vi "Fetch Multi Eval Meas List IEM Margin Results.vi"(8 "error in (no error)":errorcluster, 9 "Result Type (Current)":i32(ring) items=["Current", "Average", "Extreme", "Standard Deviation"], 10 "Instance (1)":T2=1, 11 "VISA resource name":refnum<visa-resource-name>) -> (0 "error out":errorcluster, 1 "IEM Margin Results":T1(array[cluster]) {"Carrier Leakage" format="%^.3e"; "IQ Image" format="%^.3e"; "Margin" format="%^.3e"}, 2 "Reliability":i32, 3 "VISA resource name out":refnum<visa-resource-name>)   [LabVIEW 2020, in "Rohde&Schwarz CMXP NR FR2 Measurement.lvlib"]
doc: "Returns the inband emission limit line margin results for all measured list mode segments.\n\nAttributes:\nRSCMXPNRFR2M_ATTR_FETCH_MULTI_EVAL_MEASUREMENT_LIST_IEM_MARGIN_AVERAGE_RESULTS\nRSCMXPNRFR2M_ATTR_FETCH_MULTI_EVAL_MEASUREMENT_LIST_IEM_MARGIN_CURRENT_RESULTS\nRSCMXPNRFR2M_ATTR_FETCH_MULTI_EVAL_MEASUREMENT_LIST_IEM_MARGIN_EXTREME_RESULTS\nRSCMXPNRFR2M_ATTR_FETCH_MULTI_EVAL_MEASUREMENT_LIST_IEM_MARGIN_STANDARD_DEVIATION_RESULTS\n\nRemote-control commands:\nFETCh:NRMMw:MEAS<i>:MEValuation:LIST:IEMission:MARGin:AVERage?\nFETCh:NRMMw:MEAS<i>:MEValuation:LIST:IEMission:MARGin:CURRent?\nFETCh:NRMMw:MEAS<i>:MEValuation:LIST:IEMission:MARGin:EXTReme?\nFETCh:NRMMw:MEAS<i>:MEValuation:LIST:IEMission:MARGin:SDEViation?"
uses:
  <instrlib>/Rohde&Schwarz CMXP NR FR2 Measurement/Rohde&Schwarz CMXP NR FR2 Measurement.lvlib
  <instrlib>/Rohde&Schwarz CMXP NR FR2 Measurement/Private/_Instance.ctl
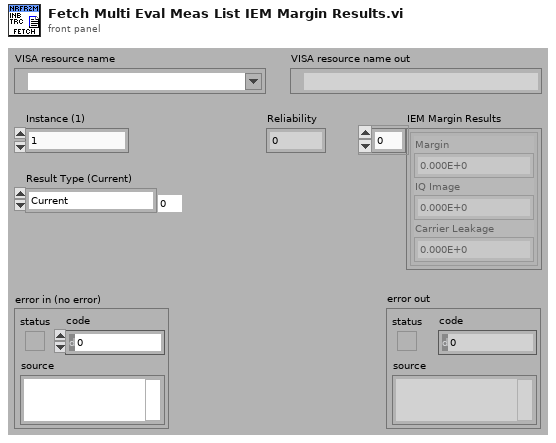
[diagram p1: front panel]
types:
  T1 = cluster{"Margin":dbl, "IQ Image":dbl, "Carrier Leakage":dbl}[]
  T2 = typedef "Rohde&Schwarz CMXP NR FR2 Measurement.lvlib/_Instance.ctl" = i32
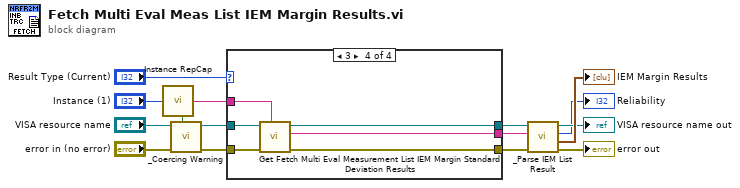
[diagram p0: block diagram]
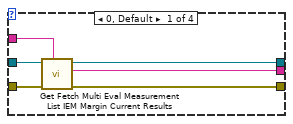
[diagram p2: hidden frame]
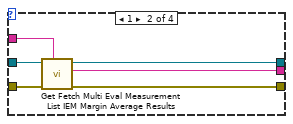
[diagram p3: hidden frame]
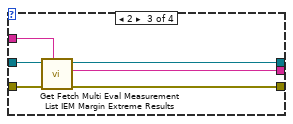
[diagram p4: hidden frame]
diagram:
  n1 = call <instrlib>:"Instance RepCap.vi"("Instance In"="Instance (1)") -> ("In Range?"=w13:bool, "RepCap Identifier Out"=w3:string)  [unwired: 1 in]
  n2 = call <instrlib>:"_Coercing Warning.vi"("In Range?"=w13, "error in (no error)"="error in (no error)", "VISA resource name"="VISA resource name") -> ("error out"=w12:errorcluster, "VISA resource name out"=w11:refnum<visa-resource-name>)  [unwired: 7 in]
  n3 = case shown="3" "Result Type (Current)" {
    tunnel: w12 -> [w21 w27 w33 w39]
    tunnel: w11 -> [w20 w26 w32 w38]
    tunnel: [w19 w25 w31 w37] -> w10
    tunnel: [w18 w24 w30 w36] -> w8
    tunnel: [w17 w23 w29 w35] -> w7
    tunnel: w3 -> [w16 w22 w28 w34]
    frame 0, Default {
      n4 = call "Get Fetch Multi Eval Measurement List IEM Margin Current Results"("Repeated Capabilities"=w16, "error in (no error)"=w21, "instrument handle"=w20) -> ("error out"=w19:errorcluster, "Fetch Multi Eval Measurement List IEM Margin Current Results"=w17:string, "instrument handle out"=w18:refnum<visa-resource-name>)  [unwired: 6 in]
    }
    frame 1 {
      n5 = call "Get Fetch Multi Eval Measurement List IEM Margin Average Results"("Repeated Capabilities"=w22, "error in (no error)"=w27, "instrument handle"=w26) -> ("error out"=w25:errorcluster, "Fetch Multi Eval Measurement List IEM Margin Average Results"=w23:string, "instrument handle out"=w24:refnum<visa-resource-name>)  [unwired: 6 in]
    }
    frame 2 {
      n6 = call "Get Fetch Multi Eval Measurement List IEM Margin Extreme Results"("Repeated Capabilities"=w28, "error in (no error)"=w33, "instrument handle"=w32) -> ("error out"=w31:errorcluster, "Fetch Multi Eval Measurement List IEM Margin Extreme Results"=w29:string, "instrument handle out"=w30:refnum<visa-resource-name>)  [unwired: 6 in]
    }
    frame 3 {
      n7 = call "Get Fetch Multi Eval Measurement List IEM Margin Standard Deviation Results"("Repeated Capabilities"=w34, "error in (no error)"=w39, "instrument handle"=w38) -> ("error out"=w37:errorcluster, "Fetch Multi Eval Measurement List IEM Margin Standard Deviation Results"=w35:string, "instrument handle out"=w36:refnum<visa-resource-name>)  [unwired: 6 in]
    }
  }
  n8 = call <instrlib>:"_Parse IEM List Result.vi"("error in (no error)"=w10, "Input String"=w7, "VISA resource name"=w8) -> ("error out"=→"error out":errorcluster, "Results"=→"IEM Margin Results":T1, "Reliability"=→"Reliability":i32, "VISA resource name out"=→"VISA resource name out":refnum<visa-resource-name>)  [unwired: 5 in]
